vi "AssertComplex_2DArray-CDB.vi"(8 "error in":errorcluster, 11 "Array":cdb[][](array[numeric])) -> (0 "error out":errorcluster, 3 "Array":cdb[][](array[numeric]))   [LabVIEW 2020, in "OpenLvVision_OpenCv.lvlib"]
uses:
  OpenLvVision_OpenCv.lvlib
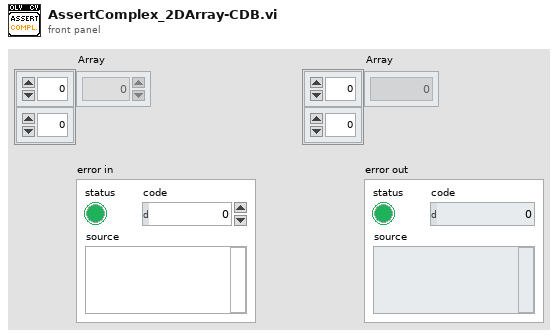
[diagram p1: front panel]
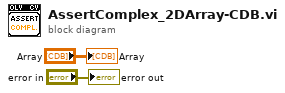
[diagram p0: block diagram]
diagram:
  "error out" <- "error in"
  "Array" <- "Array"
